vi "PracticaSemaforo.vi"() -> ()   [LabVIEW 2024]
panel:
  out "Luz roja":bool
  out "Luz amarilla":bool
  out "Luz verde":bool
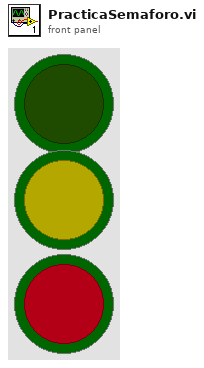
[diagram p1: front panel]
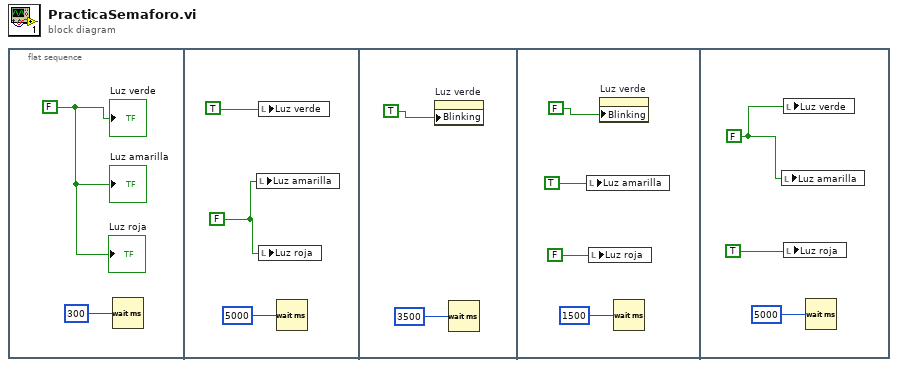
[diagram p0: block diagram]
diagram:
  n1 = flat-sequence {
    frame #0 {
      w2 = FALSE
      n2 = Wait (ms)(milliseconds to wait=u32 300 ("millisecond timer value")) -> ()  [unwired: 1 out]
      "Luz verde" <- w2
      "Luz amarilla" <- w2
      "Luz roja" <- w2
    }
    frame #1 {
      w3 = FALSE
      n3 = local write "Luz amarilla"(w3) -> ()
      n4 = local write "Luz verde"(TRUE) -> ()
      n5 = local write "Luz roja"(w3) -> ()
      n6 = Wait (ms)(milliseconds to wait=u32 5000 ("millisecond timer value")) -> ()  [unwired: 1 out]
    }
    frame #2 {
      n7 = property on="Luz verde" class="Bool (strict)"("Blinking"=TRUE) -> ()  [unwired: 2 in, 2 out]
      n8 = Wait (ms)(milliseconds to wait=u32 3500 ("millisecond timer value")) -> ()  [unwired: 1 out]
    }
    frame #3 {
      n9 = local write "Luz amarilla"(TRUE) -> ()
      n10 = local write "Luz roja"(FALSE) -> ()
      n11 = property on="Luz verde" class="Bool (strict)"("Blinking"=FALSE) -> ()  [unwired: 2 in, 2 out]
      n12 = Wait (ms)(milliseconds to wait=u32 1500 ("millisecond timer value")) -> ()  [unwired: 1 out]
    }
    frame #4 {
      w14 = FALSE
      n13 = local write "Luz amarilla"(w14) -> ()
      n14 = local write "Luz verde"(w14) -> ()
      n15 = local write "Luz roja"(TRUE) -> ()
      n16 = Wait (ms)(milliseconds to wait=u32 5000 ("millisecond timer value")) -> ()  [unwired: 1 out]
    }
  }
